vi "Create.vi"(8 "error in (no error)":errorcluster, 9 "Allow Close (T)":bool=TRUE, 10 "Plugin GUI Path":path) -> (0 "error out":errorcluster, 3 "PluginGUI out":refnum<class "PluginGUI.lvclass">)   [LabVIEW 2020, in "VolatusGUI.lvlib" / "PluginGUI.lvclass"]
uses:
  PluginGUI.lvclass
  PluginGUI.lvclass/PluginGUI.ctl
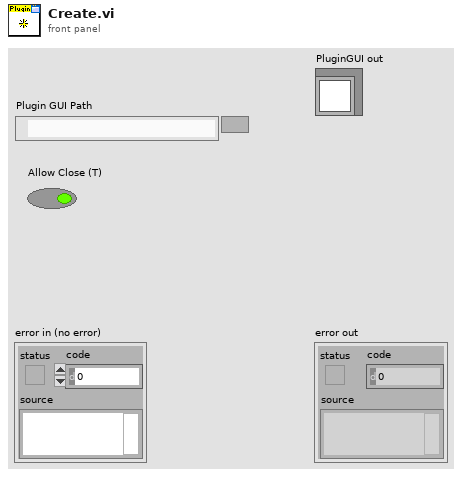
[diagram p1: front panel]
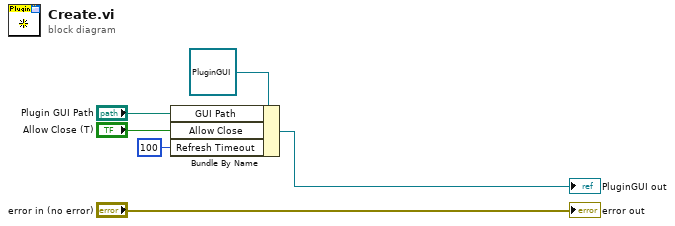
[diagram p0: block diagram]
diagram:
  n1 = Bundle By Name(cluster=refnum<class "PluginGUI.lvclass"> refnum ("PluginGUI in"), "GUI Path"="Plugin GUI Path", "Allow Close"="Allow Close (T)", "Refresh Timeout"=100) -> (→"PluginGUI out":refnum<class "PluginGUI.lvclass">)
  "error out" <- "error in (no error)"
